vi "Initialize_Robotics_Cape.vi"() -> (0 "error out":errorcluster)   [LabVIEW 2014]
uses:
  <userlib>/UCSD Robotics Lab/Robotics-Cape/LV/libroboticscape.lvlib
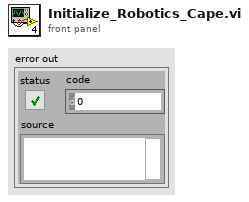
[diagram p1: front panel]
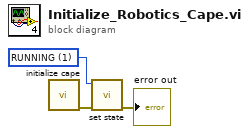
[diagram p0: block diagram]
diagram:
  w2 = u32 1 items=["UNINITIALIZED", "RUNNING", "PAUSED", "EXITING"] ("new_state")
  n1 = call <userlib>:"initialize cape.vi"() -> ("error out"=w1:errorcluster)  [unwired: 10 in, 1 out]
  n2 = call <userlib>:"set state.vi"("error in (no error)"=w1, "new_state"=w2) -> ("error out"=→"error out":errorcluster)  [unwired: 8 in, 1 out]
